vi "DontTip.vi"(11 "Motor":cluster{"Right":dbl, "Left":dbl}) -> (2 "Left":dbl, 3 "Right":dbl)   [LabVIEW 2012]
uses:
  <vilib>/ptbypt/NI_PtbyPt.lvlib
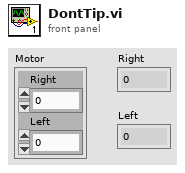
[diagram p1: front panel]
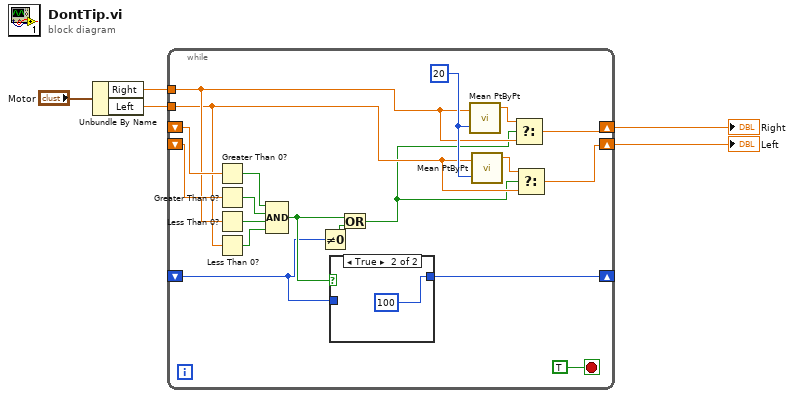
[diagram p0: block diagram]
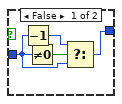
[diagram p2: hidden frame]
diagram:
  n1 = Unbundle By Name("Motor") -> ("Right"=w2:dbl, "Left"=w1:dbl)
  n2 = while {
    shift-right: [w7] -> w4
    shift-left: _ -> [w23]
    shift-right: [w8] -> w3
    shift-left: _ -> [w22]
    tunnel: w2 -> [w10]
    tunnel: w1 -> [w9]
    shift-right: [w15] -> _
    shift-left: _ -> [w14]
    stop <- TRUE stop-if-true
    w13 = 20 ("sample length")
    n3 = Greater Than 0?(x=w23) -> (x > 0?=w21:bool)
    n4 = Greater Than 0?(x=w22) -> (x > 0?=w19:bool)
    n5 = Less Than 0?(x=w10) -> (x < 0?=w18:bool)
    n6 = Less Than 0?(x=w9) -> (x < 0?=w20:bool)
    n7 = Compound Arithmetic op=AND(w21, w19, w18, w20) -> (w17:bool)
    n8 = Not Equal To 0?(x=w14) -> (x != 0?=w16:bool)
    n9 = case shown="True" w17 {
      tunnel: [w28 100] -> w15
      tunnel: w14 -> [w25 _]
      frame False {
        n10 = Decrement(x=w25) -> (x-1=w26:i32)
        n11 = Not Equal To 0?(x=w25) -> (x != 0?=w27:bool)
        n12 = Select(t=w26, s=w27, f=w25) -> (s? t:f=w28:i32)
      }
      frame True {
      }
    }
    n13 = Or(x=w17, y=w16) -> (x .or. y?=w6:bool)
    n14 = call <vilib>:"Mean PtByPt.vi"("x"=w10, "sample length"=w13) -> ("mean"=w11:dbl)  [unwired: 2 in, 1 out]
    n15 = call <vilib>:"Mean PtByPt.vi"("x"=w9, "sample length"=w13) -> ("mean"=w12:dbl)  [unwired: 2 in, 1 out]
    n16 = Select(t=w11, s=w6, f=w10) -> (s? t:f=w7:dbl)
    n17 = Select(t=w12, s=w6, f=w9) -> (s? t:f=w8:dbl)
  }
  "Left" <- w3
  "Right" <- w4
